vi "Init Msg Input.vi"(6 "Teller":refnum<class "Teller.lvclass">) -> (3 "TEMPLATE Msg Input out":refnum<class "TEMPLATE Msg Input.lvclass">)   [LabVIEW 2025, in "_Template.lvlib" / "Templates.lvlib" / "TEMPLATE jettl Msg.lvlib" / "TEMPLATE Msg Input.lvlib" / "TEMPLATE Msg Input.lvclass"]
uses:
  TEMPLATE Msg Input.lvclass
  jettl/jettl/Teller/Teller.lvclass
  TEMPLATE Msg Input.lvclass/TEMPLATE Msg Input.ctl
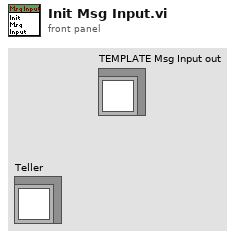
[diagram p1: front panel]
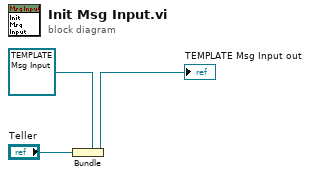
[diagram p0: block diagram]
diagram:
  n1 = Bundle "Bundle"(cluster=refnum<class "TEMPLATE Msg Input.lvclass"> refnum ("TEMPLATE Msg Input out"), "Teller") -> (→"TEMPLATE Msg Input out":refnum<class "TEMPLATE Msg Input.lvclass">)
